vi "Write Data.vi"(9 "Data":string, 11 "Save File in":refnum<class "Save File.lvclass">) -> (3 "Save File out":refnum<class "Save File.lvclass">)   [LabVIEW 2018, in "Save File Actor.lvlib" / "Save File.lvclass"]
uses:
  Save File.lvclass
  Save File.lvclass/Save File.ctl
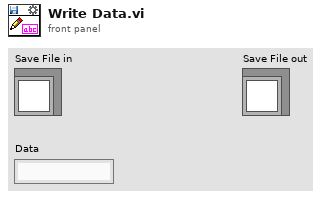
[diagram p1: front panel]
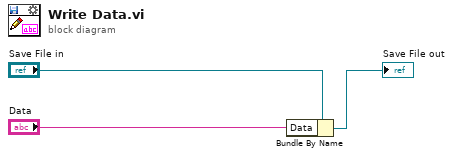
[diagram p0: block diagram]
diagram:
  n1 = Bundle By Name(cluster="Save File in", "Data"="Data") -> (→"Save File out":refnum<class "Save File.lvclass">)
